vi "20211008_HW00.vi"() -> ()   [LabVIEW 2019]
panel:
  out "Numeric":i32
  in  "Add 1":bool
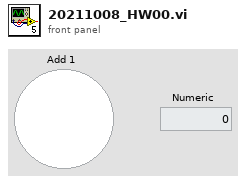
[diagram p1: front panel]
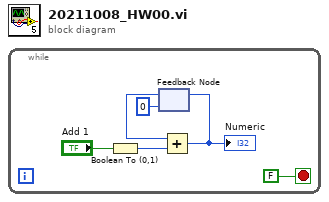
[diagram p0: block diagram]
diagram:
  n1 = while {
    stop <- FALSE stop-if-true
    n2 = Boolean To (0,1)(Boolean="Add 1") -> (0, 1=w3:i16)
    n3 = feedback #1(0) -> (w6:i32)
    n4 = Add(x=w6, y=w3) -> (x+y=w2:i32)
    "Numeric" <- w2
    n5 = feedback-in #1(w2) -> ()
  }
